vi "fgv_stop-point_databuf.vi"(7 "cmd":enum16{"clear", "write", "read"}(ring), 11 "stop pt array":cluster{dbl, dbl}[](array[cluster])) -> (3 "all stop pts out":cluster{dbl, dbl}[](array[cluster]))   [LabVIEW 2019]
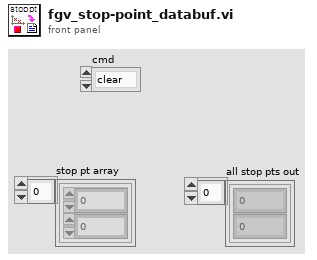
[diagram p1: front panel]
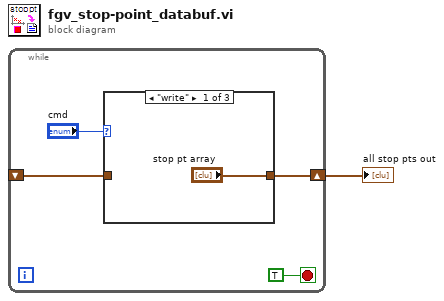
[diagram p0: block diagram]
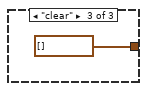
[diagram p3: hidden frame]
diagram:
  n1 = while {
    shift-right: [w3] -> w1
    shift-left: _ -> [w2]
    stop <- TRUE stop-if-true
    n2 = case shown="\"write\"" "cmd" {
      tunnel: ["stop pt array" w7 cluster{dbl, dbl}[] [] ("stop pt array")] -> w3
      tunnel: w2 -> [_ w7 _]
      frame "write" {
      }
      frame "read", Default {
      }
      frame "clear" {
      }
    }
  }
  "all stop pts out" <- w1
